vi "GlobalSettingsFGV.vi"(8 "FGVAction (Read)":T2, 11 "GlobalSettingsIn":T1={"fs [Hz]"=0.0, "Create Network Stream Timeout"=-314004, "Read Network Stream Timeout"=-314004}) -> (3 "GlobalSettingsOut":T1={"fs [Hz]"=0.0, "Create Network Stream Timeout"=-314004, "Read Network Stream Timeout"=-314004})   [LabVIEW 2019]
uses:
  FGVAction.ctl
  GlobalSettings.ctl
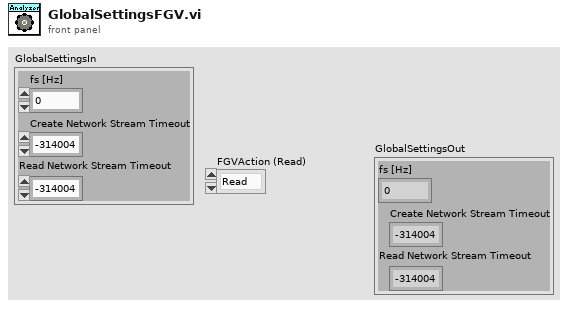
[diagram p1: front panel]
types:
  T1 = typedef "GlobalSettings.ctl" = cluster{"fs [Hz]":dbl, "Create Network Stream Timeout":i32, "Read Network Stream Timeout":i32}
  T2 = typedef "FGVAction.ctl" = enum16{"Read", "Write"}
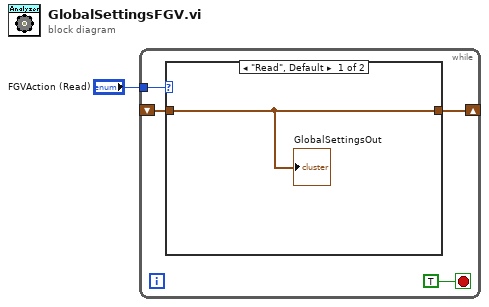
[diagram p0: block diagram]
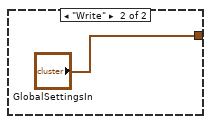
[diagram p2: hidden frame]
diagram:
  n1 = while {
    tunnel: "FGVAction (Read)" -> [w4]
    shift-right: [w2] -> _
    shift-left: _ -> [w3]
    stop <- TRUE stop-if-true
    n2 = case shown="\"Read\", Default" w4 {
      tunnel: w3 -> [w6 _]
      tunnel: [w6 "GlobalSettingsIn"] -> w2
      frame "Read", Default {
        "GlobalSettingsOut" <- w6
      }
      frame "Write" {
      }
    }
  }
